vi "CRYLoad Recnet.vi"(2 "menu tag":string) -> (0 "error out":errorcluster)   [LabVIEW 2013]
doc: "Config File Reading/Writting\n\nPath \n ini File path\nRWFlag\n 0: no action\n 1: read\n 2: write"
uses:
  CRYMainGlobal.vi
panel:
  in  "error in (no error)":errorcluster
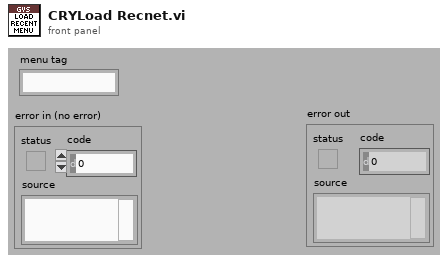
[diagram p1: front panel]
types:
  T1 = cluster{"Section":string, "Items":cluster{"Key":string, "Value":string}[]}[]
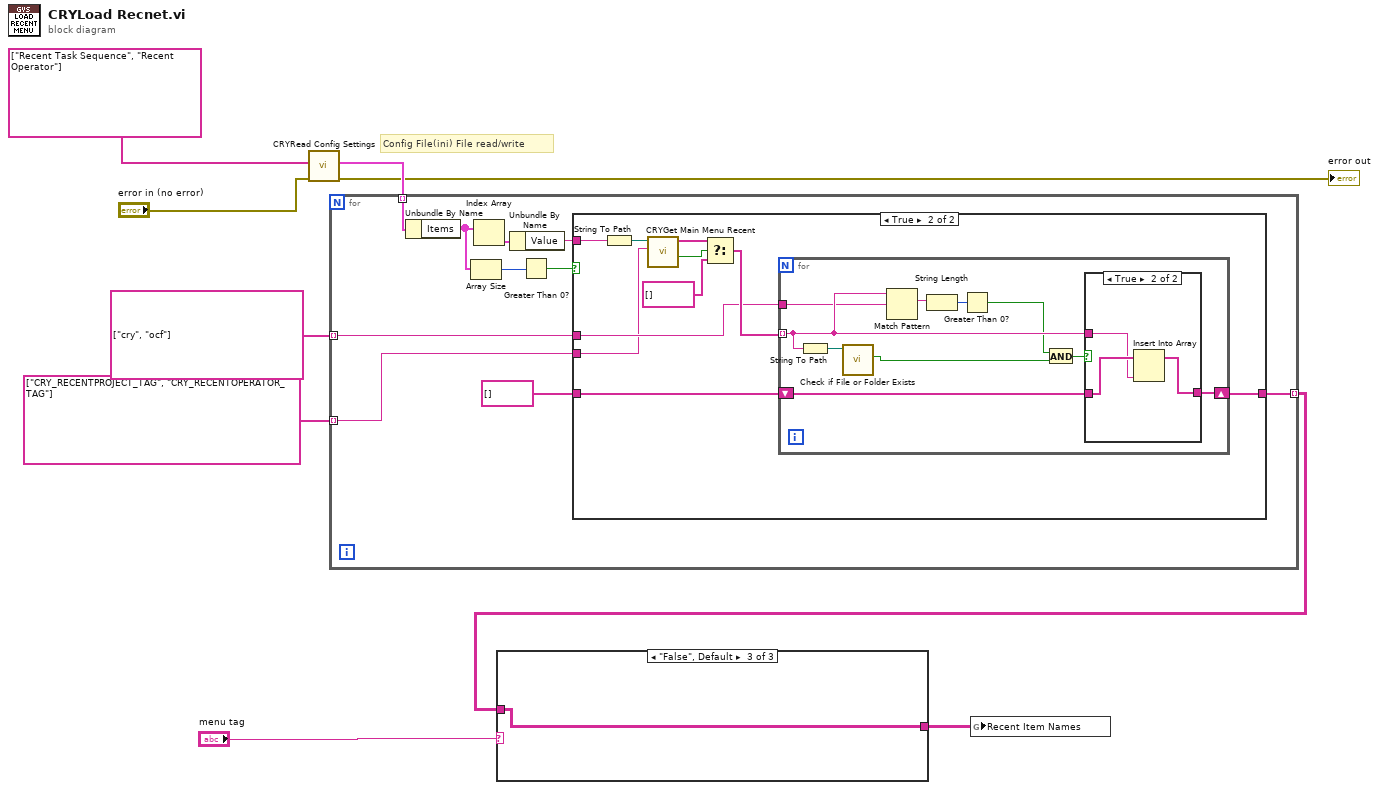
[diagram p0: block diagram]
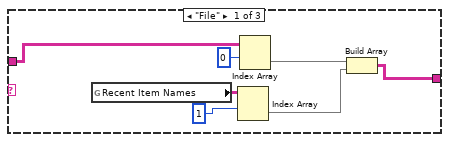
[diagram p2: hidden frame]
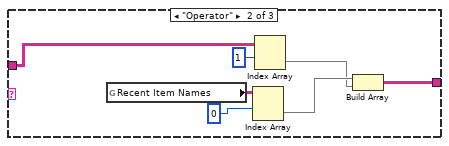
[diagram p3: hidden frame]
diagram:
  # "Config File(ini) File read/write"
  n1 = call "CRYRead Config Settings.vi"("error in (no error)"="error in (no error)", "Section"=string[] ["Recent Task Sequence", "Recent Operator"]) -> ("error out"=→"error out":errorcluster, "Configuration Data"=w8:T1)  [unwired: 8 out]
  n2 = for {
    tunnel: w8 -> [w19] mode=indexing
    tunnel: string[] ["cry", "ocf"] -> [w12] mode=indexing
    tunnel: [w11] -> w2 mode=indexing
    tunnel: string[] ["CRY_RECENTPROJECT_TAG", "CRY_RECENTOPERATOR_TAG"] -> [w10] mode=indexing
    n3 = Unbundle By Name(w19) -> ("Items"=w18:cluster{"Key":string, "Value":string}[])
    n4 = Array Size(array=w18) -> (size(s)=w17:i32)
    n5 = Index Array(array=w18) -> (element=w15:cluster{"Key":string, "Value":string})  [unwired: 1 in]
    n6 = Unbundle By Name(w15) -> ("Value"=w14:string)
    n7 = Greater Than 0?(x=w17) -> (x > 0?=w16:bool)
    n8 = case shown="True" w16 {
      tunnel: w14 -> [_ w30]
      tunnel: string[] [] ("Recent Item Names") -> [w20 w24]
      tunnel: [w20 w23] -> w11
      tunnel: w12 -> [_ w22]
      tunnel: w10 -> [_ w21]
      frame False {
      }
      frame True {
        n9 = String To Path(string=w30) -> (path=w29:path)
        n10 = call "CRYGet Main Menu Recent.vi"("Menu TAG"=w21, "RecentFiles"=w29) -> ("Seq Result"=w28:bool, "Seq Item Names Out"=w27:string[])  [unwired: 8 out]
        n11 = Select(t=w27, s=w28, f=string[] []) -> (s? t:f=w25:string[])
        n12 = for {
          tunnel: w25 -> [w37] mode=indexing
          shift-right: [w38] -> w23
          shift-left: w24 -> [w39]
          tunnel: w22 -> [w31]
          n13 = String To Path(string=w37) -> (path=w40:path)
          n14 = call <vilib>:"Check if File or Folder Exists.vi"("path"=w40) -> ("file or folder exists?"=w33:bool)  [unwired: 8 in, 2 out]
          n15 = Match Pattern(string=w37, regular expression=w31) -> (match substring=w36:string)  [unwired: 1 in, 3 out]
          n16 = String Length(string=w36) -> (length=w35:i32)
          n17 = Greater Than 0?(x=w35) -> (x > 0?=w32:bool)
          n18 = And(x=w32, y=w33) -> (x .and. y?=w34:bool)
          n19 = case shown="True" w34 {
            tunnel: w37 -> [_ w43]
            tunnel: w39 -> [w41 w44]
            tunnel: [w41 w42] -> w38
            frame False {
            }
            frame True {
              n20 = Insert Into Array(array=w44, new element=w43) -> (w42:string[])  [unwired: 1 in]
            }
          }
        }
      }
    }
  }
  n21 = case shown="\"False\", Default" "menu tag" {
    tunnel: w2 -> [w50 w55 w59]
    tunnel: [w45 w52 w59] -> w1
    frame "File" {
      n22 = global read "CRYMainGlobal.vi" "Recent Item Names"() -> (w51:string[][])
      n23 = Index Array(array=w51, index (row)=1) -> (element=w46:string[])  [unwired: 1 in]
      n24 = Index Array(array=w50, index (row)=0) -> (element=w48:string[])  [unwired: 1 in]
      n25 = Build Array(w48, w46) -> (w45:string[][])
    }
    frame "Operator" {
      n26 = global read "CRYMainGlobal.vi" "Recent Item Names"() -> (w58:string[][])
      n27 = Index Array(array=w58, index (row)=0) -> (element=w54:string[])  [unwired: 1 in]
      n28 = Index Array(array=w55, index (row)=1) -> (element=w53:string[])  [unwired: 1 in]
      n29 = Build Array(w54, w53) -> (w52:string[][])
    }
    frame "False", Default {
    }
  }
  n30 = global write "CRYMainGlobal.vi" "Recent Item Names"(w1) -> ()
